vi "HexStringToU16.vi"(0 "Input String":string, 7 "Starting Offset":i32) -> (4 "Number Out":u16)   [LabVIEW 2016]
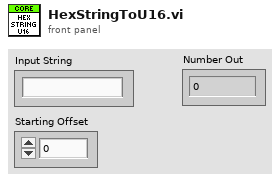
[diagram p1: front panel]
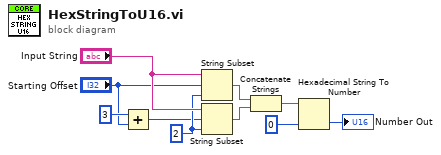
[diagram p0: block diagram]
diagram:
  w4 = 2 ("offset (0)")
  n1 = Add(x=3, y="Starting Offset") -> (x+y=w2:i32)
  n2 = String Subset(string="Input String", offset (0)="Starting Offset", length (rest)=w4) -> (substring=w8:string)
  n3 = String Subset(string="Input String", offset (0)=w2, length (rest)=w4) -> (substring=w7:string)
  n4 = Concatenate Strings(w8, w7) -> (w10:string)
  n5 = Hexadecimal String To Number(string=w10, default (0uL)=u16 0) -> (number=→"Number Out":u16)  [unwired: 1 in, 1 out]
